vi "Load Models.vi"(8 "error in (no error)":errorcluster, 9 "Models":refnum<class "Actor.lvclass">[](array[class]), 10 "Names":string[](array[string]), 11 "MVVM Abstruct Controller in":refnum<class "MVVM Abstruct Controller.lvclass">) -> (0 "error out":errorcluster, 3 "MVVM Abstruct Controller out":refnum<class "MVVM Abstruct Controller.lvclass">)   [LabVIEW 2020, in "MMVVM Framework.lvlib" / "MVVM Abstruct Controller.lvlib" / "MVVM Abstruct Controller.lvclass"]
uses:
  MVVM Abstruct Controller.lvclass
  C:/Program Files (x86)/National Instruments/LabVIEW 2020/vi.lib/ActorFramework/Actor/Actor.lvclass
  <vilib>/ActorFramework/Actor/Actor.lvclass
  MVVM Abstruct Controller.lvclass/MVVM Abstruct Controller.ctl
  ActorMap/ActorMap.lvclass
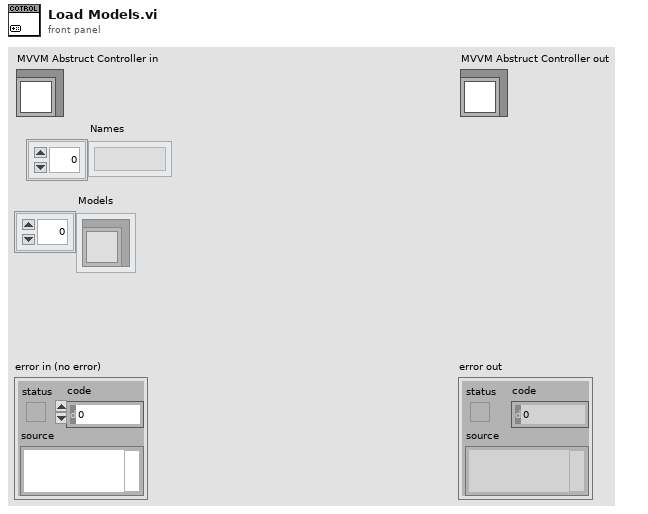
[diagram p1: front panel]
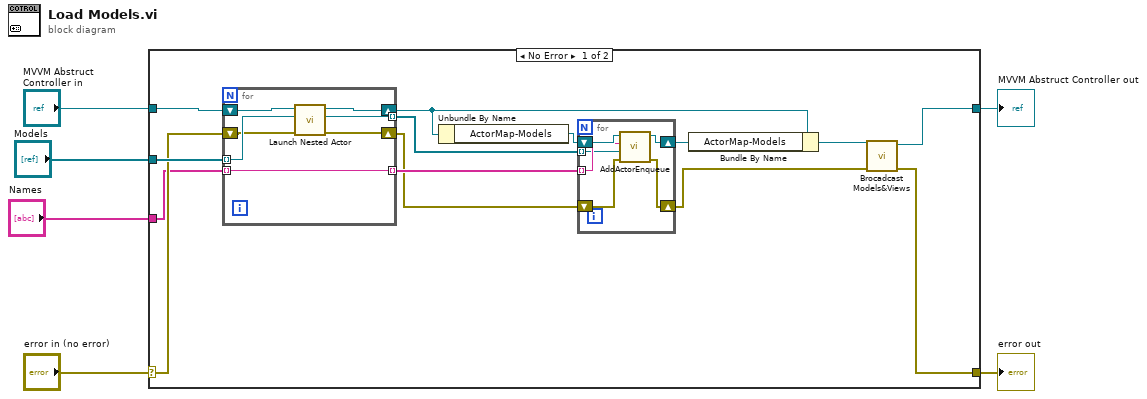
[diagram p0: block diagram]
diagram:
  n1 = case shown="No Error" "error in (no error)" {
    selector: "error in (no error)" -> [w18 w35]
    tunnel: [w7 w35] -> w5
    tunnel: [w9 w34] -> w3
    tunnel: "MVVM Abstruct Controller in" -> [w20 w34]
    tunnel: "Models" -> [w19 _]
    tunnel: "Names" -> [w17 _]
    frame No Error {
      n2 = for {
        shift-right: [w32] -> w12
        shift-left: w20 -> [w33]
        tunnel: w19 -> [w31] mode=indexing
        shift-right: [w29] -> w13
        shift-left: w18 -> [w30]
        tunnel: w17 -> [w28] mode=indexing
        tunnel: [w28] -> w15 mode=indexing
        tunnel: [w27] -> w14 mode=indexing
        n3 = call <vilib>:"Launch Nested Actor.vi"("error in (no error)"=w30, "Nested Actor"=w31, "Caller Actor in"=w33) -> ("error out"=w29:errorcluster, "Nested Actor's Enqueuer"=w27:refnum<class "Message Enqueuer.lvclass">, "Caller Actor out"=w32:refnum<class "MVVM Abstruct Controller.lvclass">)  [unwired: 6 in]
      }
      n4 = Unbundle By Name(w12) -> ("ActorMap-Models"=w16:refnum<class "ActorMap.lvclass">)
      n5 = for {
        tunnel: w15 -> [w25] mode=indexing
        tunnel: w14 -> [w24] mode=indexing
        shift-right: [w23] -> w11
        shift-left: w16 -> [w26]
        shift-right: [w21] -> w8
        shift-left: w13 -> [w22]
        n6 = call "AddActorEnqueue.vi"("error in (no error)"=w22, "Actor's Enqueuer"=w24, "name"=w25, "ActorMap in"=w26) -> ("error out"=w21:errorcluster, "ActorMap out"=w23:refnum<class "ActorMap.lvclass">)  [unwired: 6 in]
      }
      n7 = Bundle By Name(cluster=w12, "ActorMap-Models"=w11) -> (w10:refnum<class "MVVM Abstruct Controller.lvclass">)
      n8 = call "Brocadcast Models&Views.vi"("error in (no error)"=w8, "MVVM Abstruct Controller in"=w10) -> ("error out"=w7:errorcluster, "MVVM Abstruct Controller out"=w9:refnum<class "MVVM Abstruct Controller.lvclass">)  [unwired: 8 in]
    }
    frame Error {
    }
  }
  "error out" <- w5
  "MVVM Abstruct Controller out" <- w3
